vi "SENS_CORR_CSET_CRE.vi"(0 "VISA IN":refnum<visa-resource-name>, 1 "Calset":string, 5 "error in":errorcluster, 7 "Channel":i32) -> (14 "VISA Out":refnum<visa-resource-name>, 19 "error out":errorcluster)   [LabVIEW 2018, in "PNA-X.lvlib"]
doc: "SENSe<cnum>:CORRection:CSET:CREate [name] \n1690\n\n(Write-only) Creates an empty Cal Set and attaches it to the specified channel. This command is \nONLY necessary before remotely filling the Cal Set with error term data. (For Advanced Users). \nA Cal Set is automatically created, applied to the channel, and saved at the completion of a guided cal \naccording to the preference setting SENS:CORR:PREF:CSET:SAVE. \nParameters \n<cnum> Any existing channel number. If unspecified, value is set to 1 \n[name] Optional argument. Name of the Cal Set. Spaces or punctuation are NOT \nallowed. If unspecified, a unique name is chosen in the form \"Calset_N\" where \nN is a unique number. \nExamples SENS:CORR:CSET:CRE 'My2Port' \nQuery Syntax Not Applicable \nDefault Not Applicable"
uses:
  PNA-X.lvlib
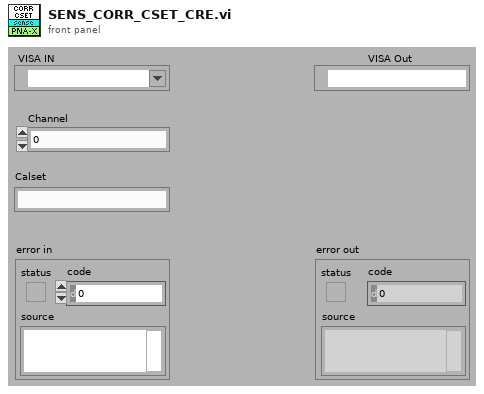
[diagram p1: front panel]
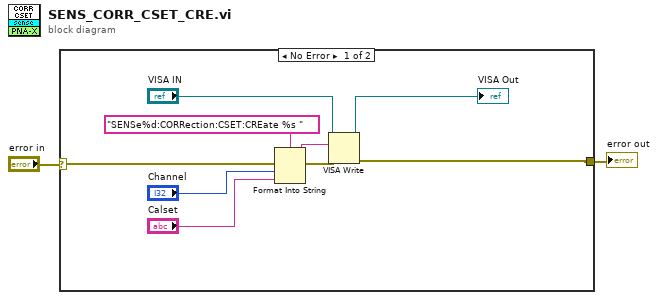
[diagram p0: block diagram]
diagram:
  n1 = case shown="No Error" "error in" {
    selector: "error in" -> [w11 w12]
    tunnel: [w6 w12] -> w1
    frame No Error {
      n2 = Format Into String(format string="SENSe%d:CORRection:CSET:CREate %s " ("Cmdline"), error in=w11, "Channel", "Calset") -> (resulting string=w9:string, error out=w10:errorcluster)  [unwired: 1 in]
      n3 = VISA Write(VISA resource name="VISA IN", write buffer=w9, error in (no error)=w10) -> (VISA resource name out=→"VISA Out":refnum<visa-resource-name>, error out=w6:errorcluster)  [unwired: 1 out]
    }
    frame Error {
    }
  }
  "error out" <- w1
